vi "Configure Average.vi"(7 "Average On":bool, 8 "error in (no error)":errorcluster, 10 "Number of Averages":i32, 11 "VNA-FieldFox in":refnum<class "VNA-FieldFox.lvclass">) -> (0 "error out":errorcluster, 3 "VNA-FieldFox out":refnum<class "VNA-FieldFox.lvclass">)   [LabVIEW 2020, in "VNA-FieldFox.lvclass"]
doc: "Configures the average to use for the sweep"
uses:
  VNA-FieldFox.lvclass
  C:/Sandbox/RF Bench/Source Code/WiSpry Test Framework/Instruments/Instrument.lvclass
  Instrument.lvclass/Instrument.ctl
  Instrument.lvclass
  <instrlib>/Agilent N99XX Series/Agilent N99XX Series.lvlib
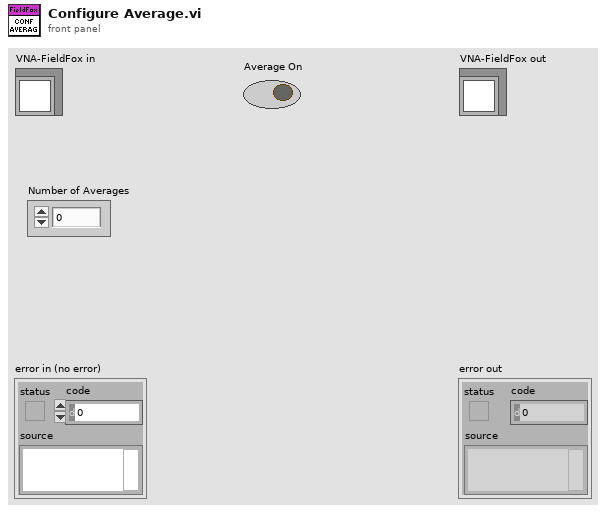
[diagram p1: front panel]
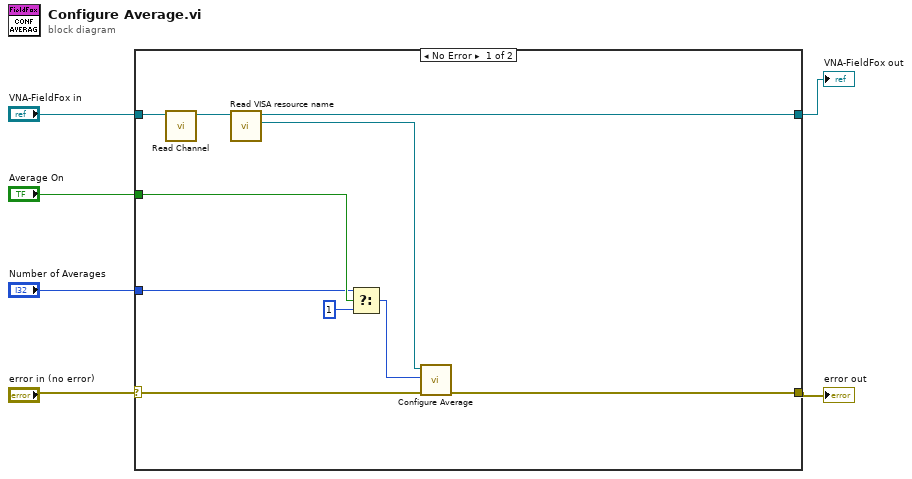
[diagram p0: block diagram]
diagram:
  n1 = case shown="No Error" "error in (no error)" {
    selector: "error in (no error)" -> [w15 w18]
    tunnel: [w14 w18] -> w1
    tunnel: [w16 w17] -> w2
    tunnel: "VNA-FieldFox in" -> [w11 w17]
    tunnel: "Number of Averages" -> [w9 _]
    tunnel: "Average On" -> [w10 _]
    frame No Error {
      n2 = call-dynamic "Read Channel.vi"("Vector Network Analyzer in"=w11) -> ("Vector Network Analyzer out"=w12:refnum<class "VNA-FieldFox.lvclass">)  [unwired: 9 in, 1 out]
      n3 = call "Read VISA resource name.vi"("Instrument in"=w12) -> ("VISA resource name"=w13:refnum<visa-resource-name>, "Instrument out"=w16:refnum<class "VNA-FieldFox.lvclass">)  [unwired: 9 in]
      n4 = Select(t=w9, s=w10, f=1) -> (s? t:f=w8:i32)
      n5 = call <instrlib>:"Configure Average.vi"("error in (no error)"=w15, "Average Count (1)"=w8, "VISA resource name"=w13) -> ("error out"=w14:errorcluster)  [unwired: 7 in, 1 out]
    }
    frame Error {
    }
  }
  "error out" <- w1
  "VNA-FieldFox out" <- w2
